vi "Old_Ref1.vi"() -> ()   [LabVIEW 2020]
doc: "This example illustrates how to transfer the current waveform on an oscilloscope using the following steps:\n\n1. Specify a valid VISA session. \n2. Specify a channel. \n3. Specify a time-out value for reading waveform.\n4. Run the VI. The graph displays the waveform you acquire."
uses:
  <instrlib>/Tektronix DPO MSO 2000 4000 Series/Public/Data/Data_Low Level/Fetch Waveform (Waveform Data Type).vi
  <vilib>/measure/mascope.llb/Transition Measurements 1 chan.vi
  <vilib>/measure/mamon.llb/Trigger Detection for 1 Channel.vi
  <instrlib>/Tektronix DPO MSO 2000 4000 Series/Tektronix DPO MSO 2000 4000 Series.lvlib
  <vilib>/measure/NI_MAPro.lvlib
panel:
  out "t0 - Channel 3":timestamp
  out "dt - Channel 3":dbl
  out "Y - Channel 3":dbl[](array[numeric])
  out "t0 - Channel 2":timestamp
  out "dt - Channel 2":dbl
  out "Y - Channel 2":dbl[](array[numeric])
  out "t0 - Channel 1":timestamp
  out "dt - Channel 1":dbl
  out "Y - Channel 1":dbl[](array[numeric])
  in  "Math":u16(ring)=4 items=["Channel 1", "Channel 2", "Channel 3", "Channel 4", "Math", "Reference 1", "Reference 2", "Reference 3", "Reference 4", "D0", "D1", "D2", "D3", "D4", "D5", "D6", "D7", "D8", "D9", "D10", "D11", "D12", "D13", "D14", "D15", "Amplitude", "Frequency", "Phase", "Normal", "Average", "Maximum Peak Hold", "Minimum Peak Hold"]
  in  "Channel 3":u16(ring)=2 items=["Channel 1", "Channel 2", "Channel 3", "Channel 4", "Math", "Reference 1", "Reference 2", "Reference 3", "Reference 4", "D0", "D1", "D2", "D3", "D4", "D5", "D6", "D7", "D8", "D9", "D10", "D11", "D12", "D13", "D14", "D15", "Amplitude", "Frequency", "Phase", "Normal", "Average", "Maximum Peak Hold", "Minimum Peak Hold"]
  in  "Channel 2":u16(ring)=1 items=["Channel 1", "Channel 2", "Channel 3", "Channel 4", "Math", "Reference 1", "Reference 2", "Reference 3", "Reference 4", "D0", "D1", "D2", "D3", "D4", "D5", "D6", "D7", "D8", "D9", "D10", "D11", "D12", "D13", "D14", "D15", "Amplitude", "Frequency", "Phase", "Normal", "Average", "Maximum Peak Hold", "Minimum Peak Hold"]
  in  "Channel 1":u16(ring) items=["Channel 1", "Channel 2", "Channel 3", "Channel 4", "Math", "Reference 1", "Reference 2", "Reference 3", "Reference 4", "D0", "D1", "D2", "D3", "D4", "D5", "D6", "D7", "D8", "D9", "D10", "D11", "D12", "D13", "D14", "D15", "Amplitude", "Frequency", "Phase", "Normal", "Average", "Maximum Peak Hold", "Minimum Peak Hold"]
  in  "Maximum Time (10000ms)":u32=10000
  in  "VISA Resource Name":refnum<visa-resource-name>
  out "Waveform Graph":waveform(dbl)[](graph)
  # "(C) 2006 - 2019. National Instruments Corporation. ALL RIGHTS RESERVED."
  # "--------------------------CHANNEL 1---------------------------"
  # "--------------------------CHANNEL 2---------------------------"
  # "--------------------------CHANNEL 3---------------------------"
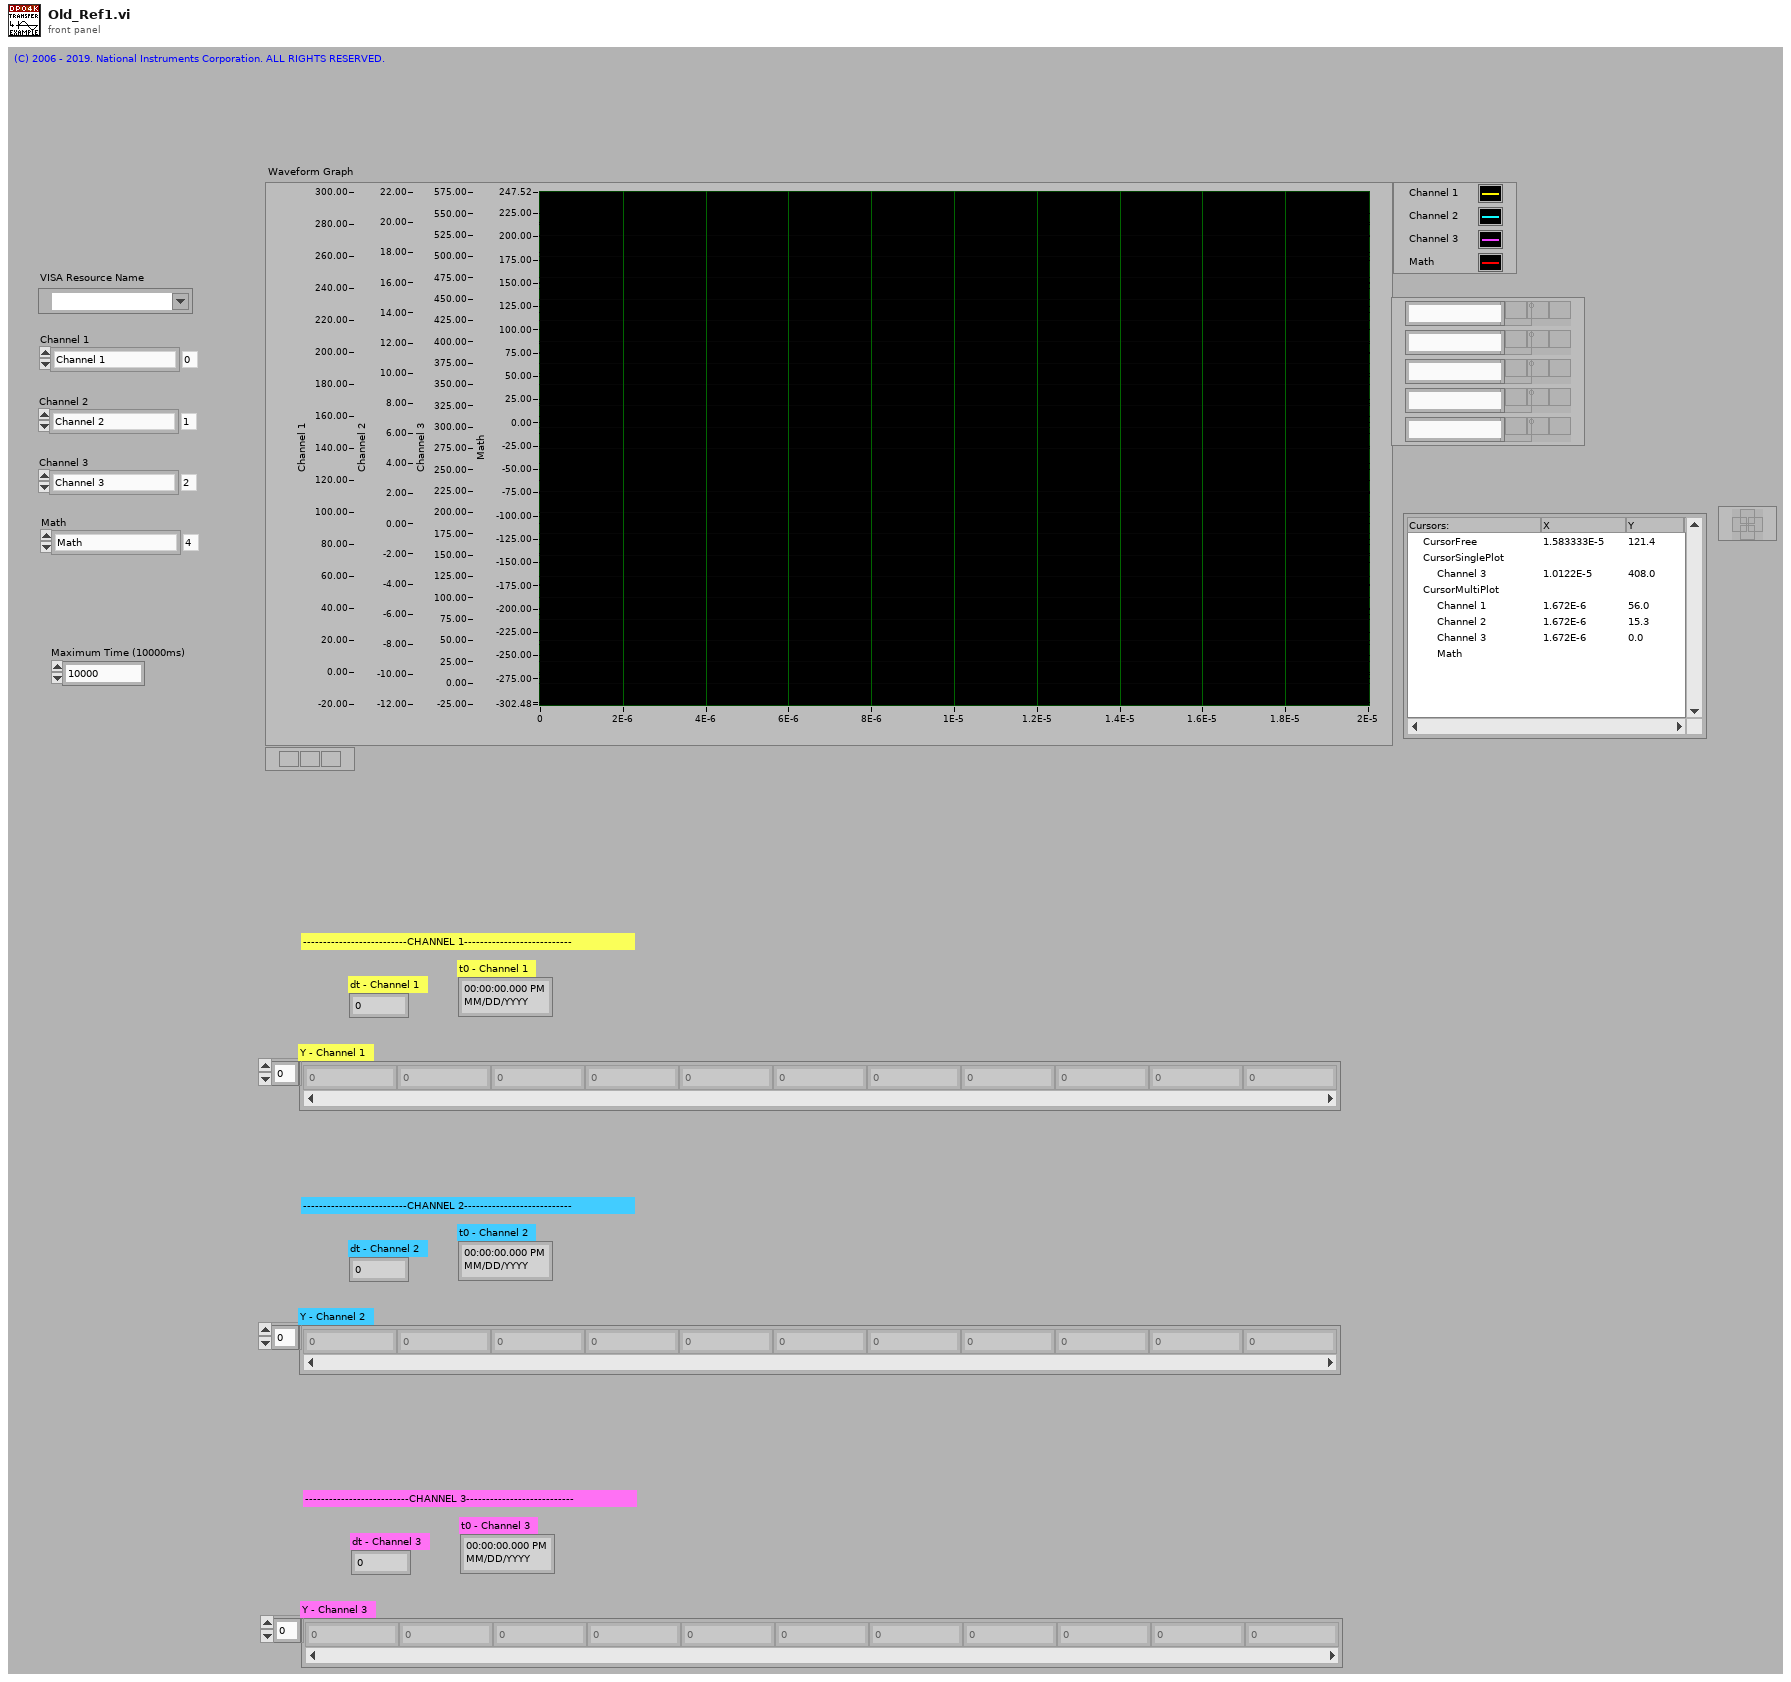
[diagram p1: front panel]
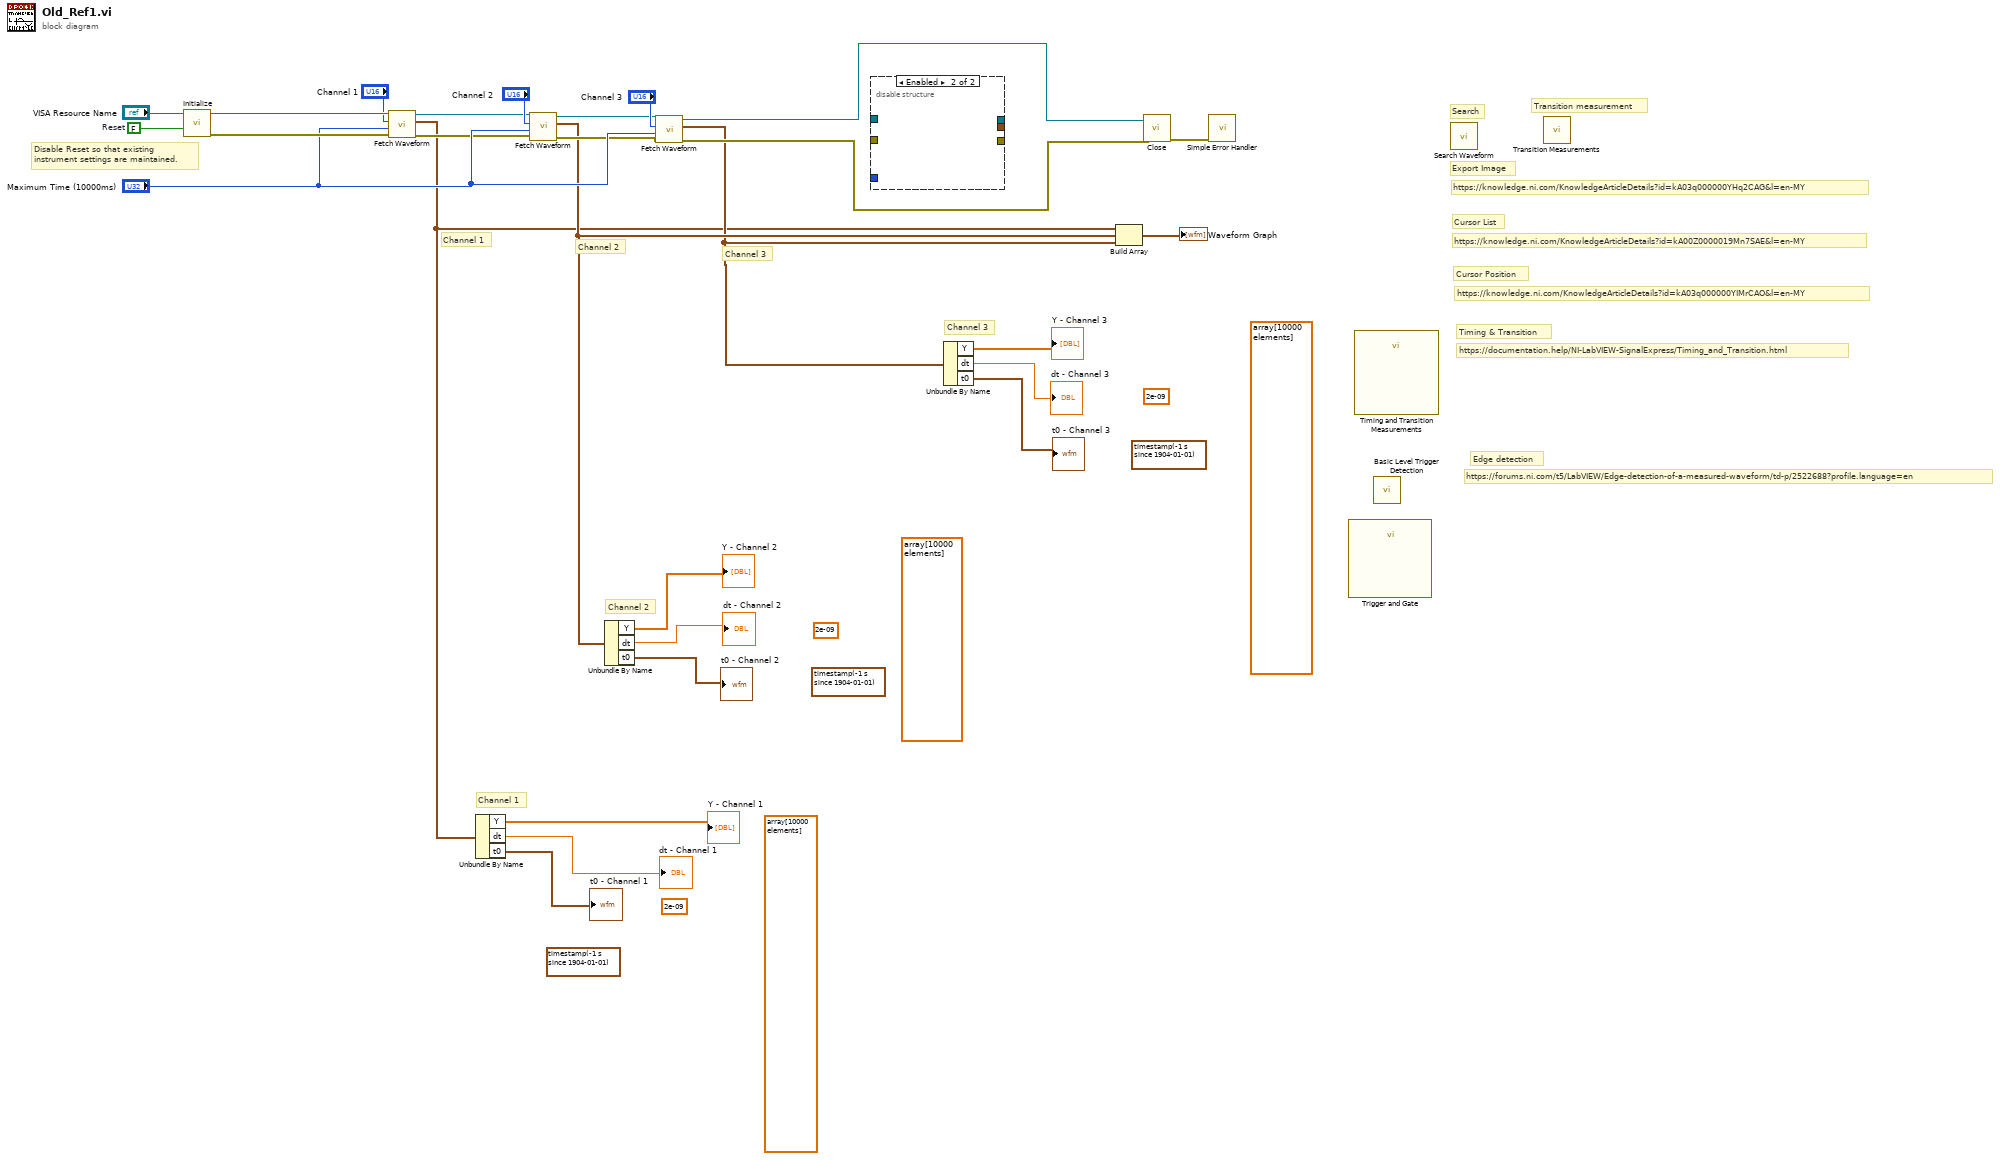
[diagram p0: block diagram]
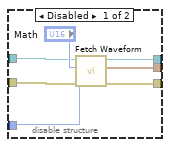
[diagram p2: hidden frame]
diagram:
  (unwired) dbl[] array[10000 elements] ("Y - Channel 3")
  (unwired) timestamp(-7.120000000027105e-06 s since 1904-01-01) ("t0 - Channel 3")
  (unwired) 2e-09 ("dt - Channel 3")
  (unwired) dbl[] array[10000 elements] ("Y - Channel 2")
  (unwired) timestamp(-7.120000000027105e-06 s since 1904-01-01) ("t0 - Channel 2")
  (unwired) 2e-09 ("dt - Channel 2")
  (unwired) dbl[] array[10000 elements] ("Y - Channel 1")
  (unwired) timestamp(-7.120000000027105e-06 s since 1904-01-01) ("t0 - Channel 1")
  (unwired) 2e-09 ("dt - Channel 1")
  w26 = FALSE  # Reset
  # "Edge detection"
  # "https://forums.ni.com/t5/LabVIEW/Edge-detection-of-a-measured-waveform/td-p/2522688?profile.language=en"
  # "https://documentation.help/NI-LabVIEW-SignalExpress/Timing_and_Transition.html"
  # "Timing & Transition"
  # "Transition measurement"
  # "Cursor Position"
  # "https://knowledge.ni.com/KnowledgeArticleDetails?id=kA03q000000YIMrCAO&l=en-MY"
  # "https://knowledge.ni.com/KnowledgeArticleDetails?id=kA00Z0000019Mn7SAE&l=en-MY"
  # "Cursor List"
  # "Export Image"
  # "https://knowledge.ni.com/KnowledgeArticleDetails?id=kA03q000000YHq2CAG&l=en-MY"
  # "Search"
  # "Channel 3"
  # "Channel 2"
  # "Channel 3"
  # "Channel 2"
  # "Channel 1"
  # "Channel 1"
  # "Disable Reset so that existing\ninstrument settings are maintained."
  n1 = call <instrlib>:"Initialize.vi"("Reset (True)"=w26, "VISA resource name"="VISA Resource Name") -> ("error out"=w24:errorcluster, "VISA resource name out"=w25:refnum<visa-resource-name>)  [unwired: 8 in]
  n2 = call-poly <instrlib>:"Fetch Waveform.vi"("error in (no error)"=w24, "Maximum Time (10000ms)"="Maximum Time (10000ms)", "Channel (0: Channel 1)"="Channel 1", "VISA resource name"=w25) -> ("error out"=w19:errorcluster, "Waveform Data"=w7:waveform(dbl), "VISA resource name out"=w18:refnum<visa-resource-name>)  [unwired: 5 in]
  n3 = Unbundle By Name(w7) -> ("Y"=→"Y - Channel 1":dbl[], "dt"=→"dt - Channel 1":dbl, "t0"=→"t0 - Channel 1":timestamp)
  n4 = call-poly <instrlib>:"Fetch Waveform.vi"("error in (no error)"=w19, "Maximum Time (10000ms)"="Maximum Time (10000ms)", "Channel (0: Channel 1)"="Channel 2", "VISA resource name"=w18) -> ("error out"=w17:errorcluster, "Waveform Data"=w12:waveform(dbl), "VISA resource name out"=w16:refnum<visa-resource-name>)  [unwired: 5 in]
  n5 = Unbundle By Name(w12) -> ("Y"=→"Y - Channel 2":dbl[], "dt"=→"dt - Channel 2":dbl, "t0"=→"t0 - Channel 2":timestamp)
  n6 = call-poly <instrlib>:"Fetch Waveform.vi"("error in (no error)"=w17, "Maximum Time (10000ms)"="Maximum Time (10000ms)", "Channel (0: Channel 1)"="Channel 3", "VISA resource name"=w16) -> ("error out"=w14:errorcluster, "Waveform Data"=w11:waveform(dbl), "VISA resource name out"=w15:refnum<visa-resource-name>)  [unwired: 5 in]
  n7 = disable-structure shown="Enabled" {
    disable-tunnel: _ -> [w34 _]
    disable-tunnel: _ -> [w33 _]
    disable-tunnel: _ -> [w32 _]
    disable-tunnel: [w31 _] -> _
    disable-tunnel: [w30 _] -> _
    disable-tunnel: [w29 _] -> _
    frame Disabled {
      n8 = call-poly <instrlib>:"Fetch Waveform.vi"("error in (no error)"=w33, "Maximum Time (10000ms)"=w34, "Channel (0: Channel 1)"="Math", "VISA resource name"=w32) -> ("error out"=w31:errorcluster, "Waveform Data"=w29:waveform(dbl), "VISA resource name out"=w30:refnum<visa-resource-name>)  [unwired: 5 in]
    }
    frame Enabled {
    }
  }
  n9 = Unbundle By Name(w11) -> ("Y"=→"Y - Channel 3":dbl[], "dt"=→"dt - Channel 3":dbl, "t0"=→"t0 - Channel 3":timestamp)
  n10 = Build Array(w7, w12, w11) -> (→"Waveform Graph":waveform(dbl)[])
  n11 = call <instrlib>:"Close.vi"("error in (no error)"=w14, "VISA resource name"=w15) -> ("error out"=w27:errorcluster)  [unwired: 9 in]
  n12 = call <vilib>:"Simple Error Handler.vi"("error in (no error)"=w27) -> ()  [unwired: 4 in, 5 out]
  n13 = call "Trigger and Gate"() -> ()  [unwired: 8 in, 4 out]
  n14 = call "Timing and Transition Measurements"() -> ()  [unwired: 11 in, 1 out]
  n15 = call-poly <vilib>:"Basic Level Trigger Detection.vi"() -> ()  [unwired: 13 in, 3 out]
  n16 = call <vilib>:"Search Waveform.vi"() -> ()  [unwired: 6 in, 6 out]
  n17 = call-poly <vilib>:"Transition Measurements.vi"() -> ()  [unwired: 6 in, 6 out]
